vi "String.Select High or Low Item form Str Array.vi"(10 "Lowest(F)/Highest(T)":bool, 11 "File Names":string[](array[string])) -> (3 "Selection":string)   [LabVIEW 2019]
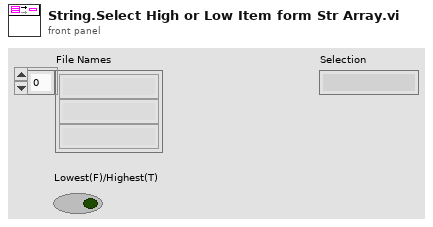
[diagram p1: front panel]
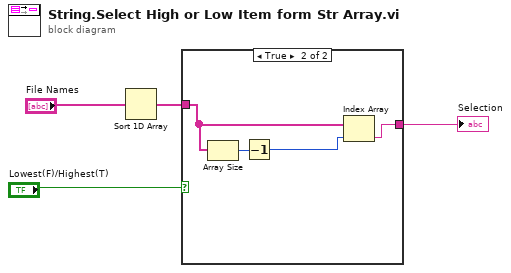
[diagram p0: block diagram]
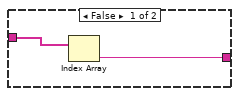
[diagram p2: hidden frame]
diagram:
  n1 = Sort 1D Array(array="File Names") -> (sorted array=w3:string[])
  n2 = case shown="True" "Lowest(F)/Highest(T)" {
    tunnel: w3 -> [w6 w8]
    tunnel: [w5 w7] -> w2
    frame False {
      n3 = Index Array(array=w6) -> (element=w5:string)  [unwired: 1 in]
    }
    frame True {
      n4 = Array Size(array=w8) -> (size(s)=w10:i32)
      n5 = Decrement(x=w10) -> (x-1=w9:i32)
      n6 = Index Array(array=w8, index=w9) -> (element=w7:string)
    }
  }
  "Selection" <- w2
